vi "Global_SM Write_Data Out.vi"() -> ()   [LabVIEW 2017, in "Claw_Rotation.lvlib"]
uses:
  startup.rtexe/Claw_Rotation.lvlib
  startup.rtexe/CLUSTER_TalonInput.ctl
  startup.rtexe/CTRE_Phoenix_MotorControl_ControlMode.ctl
  startup.rtexe/CLUSTER_PID.ctl
  ENUM_SM_State.ctl
panel:
  in  "Claw_Rotation_SM_State":T1
  in  "Claw_Rotation_SM_Output":T2 {"Talon Mode" items=["PercentOutput"=0, "Position"=1, "Velocity"=2, "Current"=3, "Follower"=5, "MotionProfile"=6, "MotionMagic"=7, "MotionMagicArc"=8, "MotionProfileArc"=10, "Disabled"=15]}
  # "The Names of the Data items in the Global Variable MUST describe who the Single Writer is\nNaming Convention of all Data Items is:   \nLib Name_Loop Name (SM or SEN or ACT)_Data Name\nExamples:\nDrive_ACT_X axis\nGameController_SEN_JoystickLeft\nHopper_SM_AgitatorSpeed"
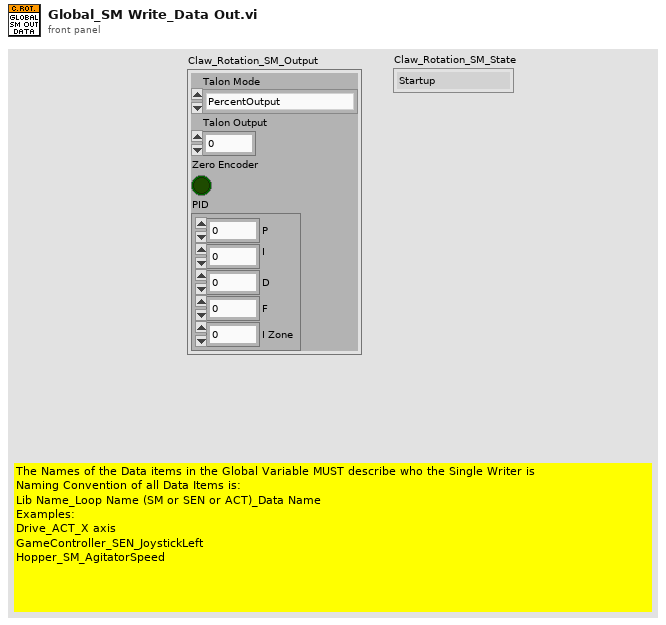
[diagram p1: front panel]
types:
  T1 = typedef "Claw_Rotation.lvlib/ENUM_SM_State.ctl" = enum16{"Startup", "Idle", "Manual", "Position - Moving", "Position - Holding", "Shutdown"}
  T2 = typedef "CLUSTER_TalonInput.ctl" = cluster{"Talon Mode":T3, "Talon Output":dbl, "Zero Encoder":bool, "PID":T4}
  T3 = typedef "CTRE_Phoenix_MotorControl_ControlMode.ctl" = u16
  T4 = typedef "CLUSTER_PID.ctl" = cluster{"P":dbl, "I":dbl, "D":dbl, "F":dbl, "I Zone":dbl}
diagram:
